vi "Communication Handler.vi"(8 "error in":errorcluster, 11 "Message Queues in":T1) -> (0 "error out":errorcluster)   [LabVIEW 2018]
uses:
  support/Message Queue/All Message Queues.ctl
  support/Message Queue/Message Cluster.ctl
  Real-Time/controls/Controller Data.ctl
  support/Message Queue/Enqueue Message (Single).vi
  support/Message Queue/Message Queue.lvlib
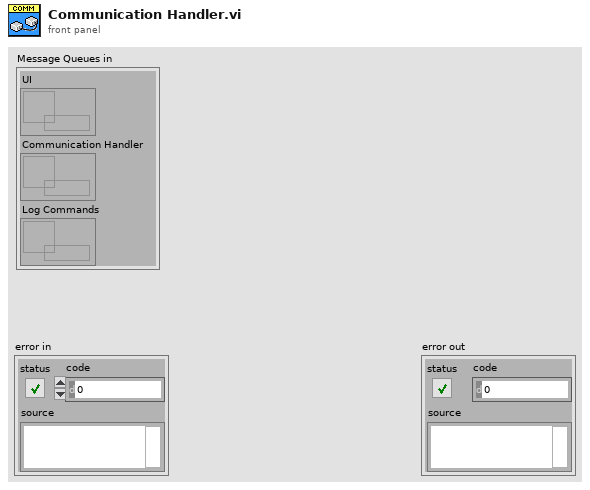
[diagram p1: front panel]
types:
  T1 = typedef "Message Queue.lvlib/All Message Queues.ctl" = cluster{"UI":refnum<queue>, "Communication Handler":refnum<queue>, "Log Commands":refnum<queue>}
  T2 = typedef "Controller Data.ctl" = cluster{"Closed Loop Enabled":bool, "Proportional valve 1":dbl, "Proportional valve 2":dbl, "Plant Control Variables":cluster{"Tank 1 Level":dbl, "Tank 2 Level":dbl, "Tank 3 Level":dbl, "Tank 4 Level":dbl, "Pump 1":dbl, "Pump 2":dbl}, "Setpoints":cluster{"Setpoint tank 1":dbl, "Setpoint tank 2":dbl}, "Controller":cluster{"A":dbl[][], "B":dbl[][], "C":dbl[][], "D":dbl[][]}}
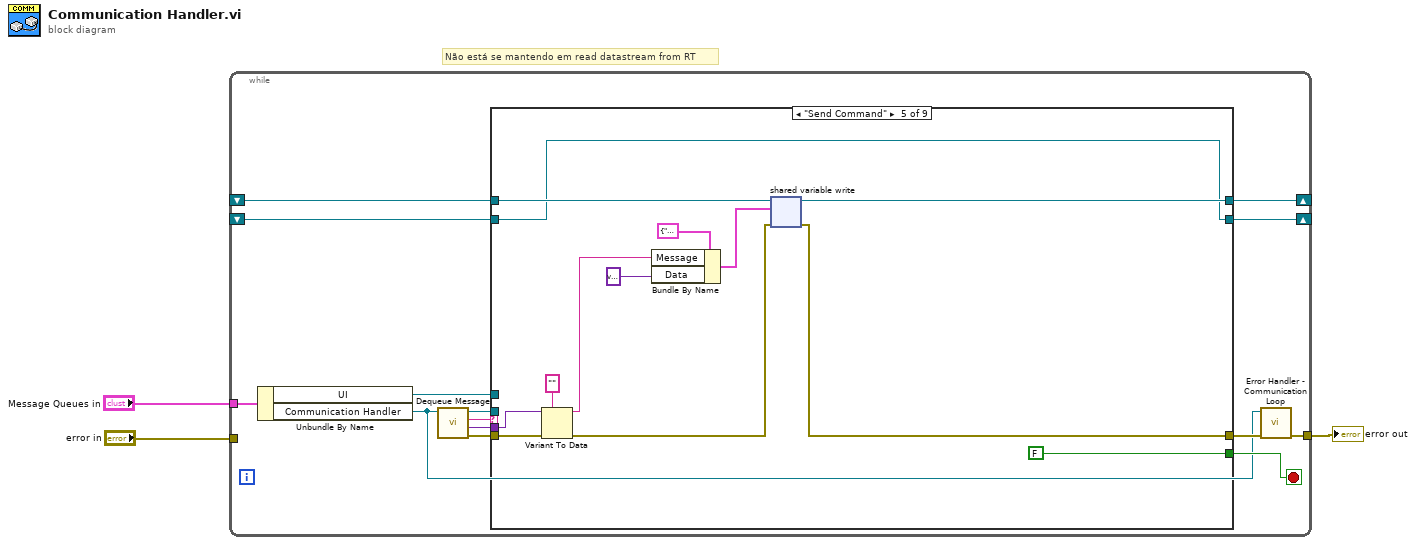
[diagram p0: block diagram]
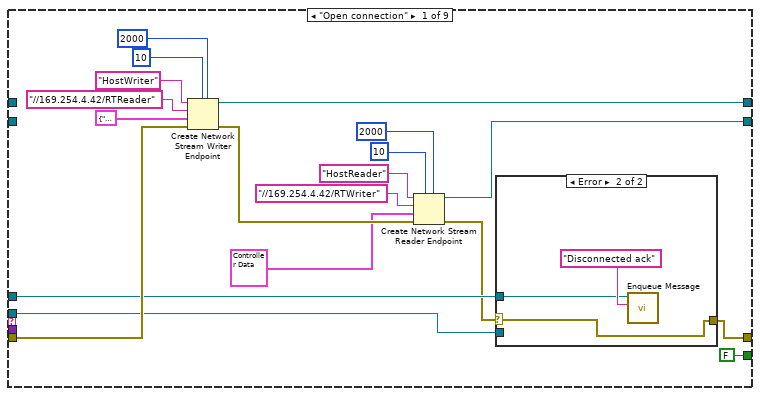
[diagram p2: hidden frame]
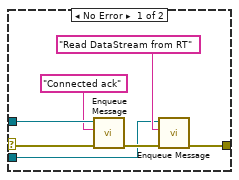
[diagram p3: hidden frame]
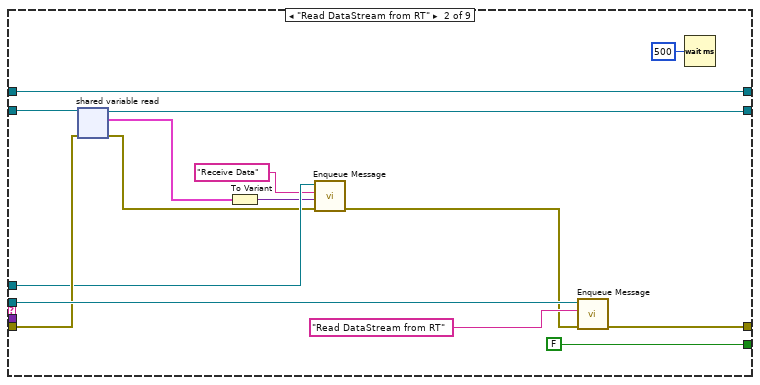
[diagram p4: hidden frame]
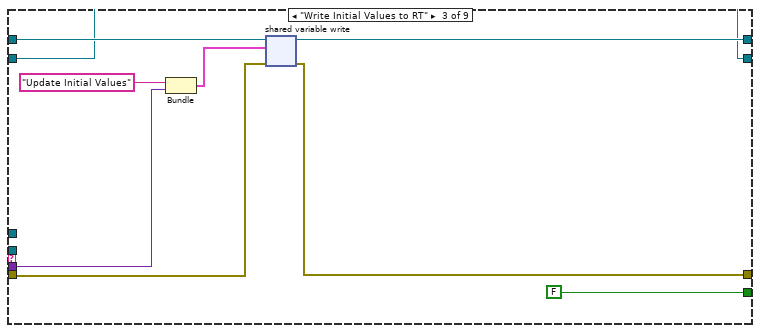
[diagram p5: hidden frame]
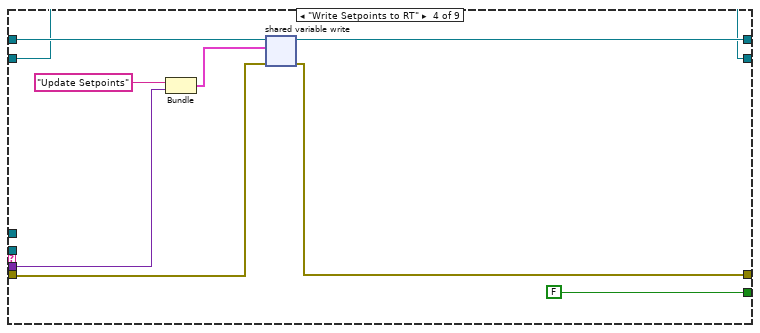
[diagram p6: hidden frame]
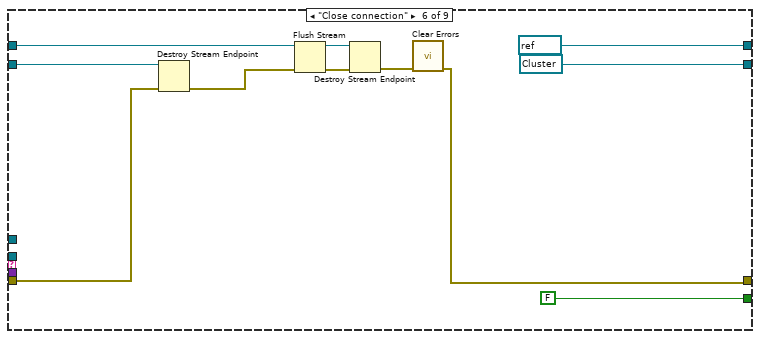
[diagram p7: hidden frame]
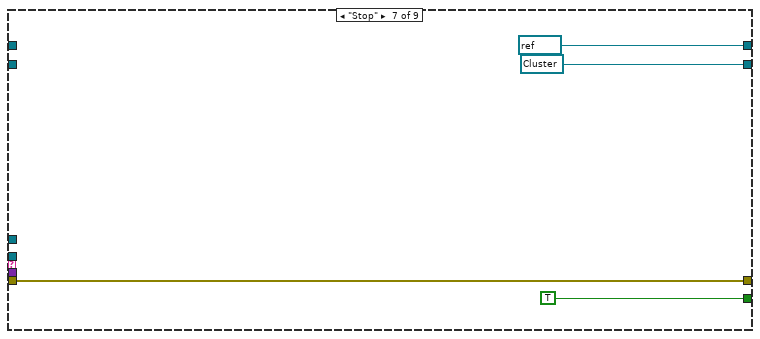
[diagram p8: hidden frame]
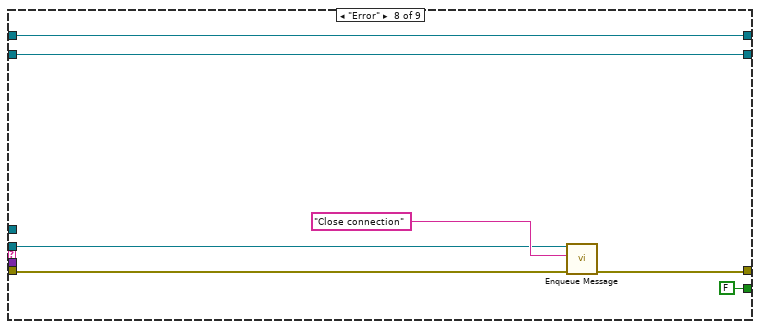
[diagram p9: hidden frame]
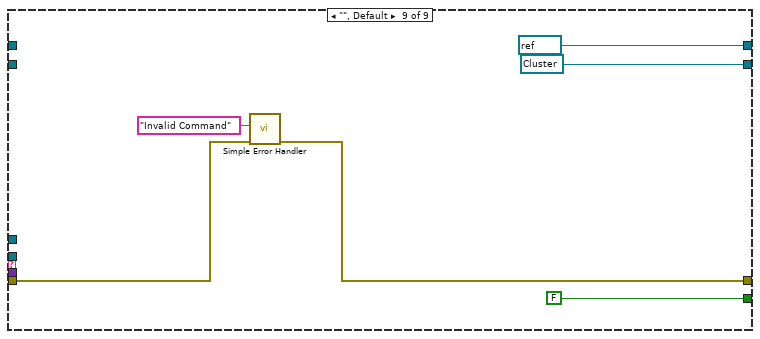
[diagram p10: hidden frame]
diagram:
  # "Não está se mantendo em read datastream from RT"
  n1 = while {
    tunnel: "Message Queues in" -> [w16]
    tunnel: [w6] -> w3
    tunnel: "error in" -> [_]
    shift-right: [w11] -> _
    shift-left: _ -> [w10]
    shift-right: [w4] -> _
    shift-left: _ -> [w9]
    stop <- w12 stop-if-true
    n2 = Unbundle By Name(w16) -> ("UI"=w15:refnum<queue>, "Communication Handler"=w5:refnum<queue>)
    n3 = call "Dequeue Message.vi"("Message Queue"=w5) -> ("error out"=w13:errorcluster, "Message Data"=w8:variant, "Message"=w17:string, "dup Message Queue"=w14:refnum<queue>)  [unwired: 7 in]
    n4 = case shown="\"Send Command\"" w17 {
      tunnel: w15 -> [w29 w56 _ _ _ _ _ _ _]
      tunnel: w14 -> [w20 w58 _ _ _ _ _ w112 _]
      tunnel: w13 -> [w30 w57 w66 w75 w86 w98 w105 w113 w120]
      tunnel: [w22 w60 w63 w72 w89 w94 w105 w109 w118] -> w7
      tunnel: [FALSE FALSE FALSE FALSE FALSE FALSE TRUE FALSE FALSE] -> w12
      tunnel: [w27 w51 w68 w77 w90 refnum<k21> refnum ("writer name") refnum<k21> refnum ("writer name") w111 refnum<k21> refnum ("writer name")] -> w11
      tunnel: w10 -> [_ w51 w69 w78 w91 w102 _ w111 _]
      tunnel: w9 -> [_ w49 w62 w71 w80 w96 _ w108 _]
      tunnel: w8 -> [_ _ w65 w74 w87 _ _ _ _]
      tunnel: [w18 w47 w62 w71 w80 refnum<k21> refnum ("writer name") refnum<k21> refnum ("writer name") w108 refnum<k21> refnum ("writer name")] -> w4
      frame "Open connection" {
        n5 = Create Network Stream Writer Endpoint(5:2000 ("timeout in ms (-1)"), 7:10 ("writer buffer size"), 8:w30, 9:cluster{string, variant} {"", variant}, 10:"//169.254.4.42/RTReader" ("writer url"), 11:"HostWriter" ("writer name")) -> (0:w31:errorcluster, 3:w27:refnum<k21>)  [unwired: 1 in]
        n6 = Create Network Stream Reader Endpoint(5:2000 ("timeout in ms (-1)"), 7:10 ("writer buffer size"), 8:w31, 9:T2 {"Closed Loop Enabled"=FALSE, "Proportional valve 1"=0.0, "Proportional valve 2"=0.0, "Plant Control Variables"={"Tank 1 Level"=0.0, "Tank 2 Level"=0.0, "Tank 3 Level"=0.0, "Tank 4 Level"=0.0, "Pump 1"=0.0, "Pump 2"=0.0}, "Setpoints"={"Setpoint tank 1"=0.0, "Setpoint tank 2"=0.0}, "Controller"={"A"=[[-4.94989, 0.0218181, -352.966, 23.8192, -3.10685, -0.000952287], [-0.0218181, -4.904857, 23.4819, -343.472, 0.000977323, -3.58066], [0.0389045, 0.0, -31.6573, 0.0287797, 0.0245405, 0.0], [0.0, 0.0381972, 0.0287797, -31.6573, 0.0, 0.0280468], [0.0, 0.0325383, 0.0240248, -0.0293675, -0.0245405, 0.0], [0.031831, 0.0, -0.0282058, 0.0, 0.0, 0.0]], "B"=[[28.0692, -23.9099], [-23.3912, 28.5852], [31.6468, -0.0287797], [-0.0287797, 31.6468], [-0.0282058, -0.0293675], [0.0282058, -0.0240214]], "C"=[[4.94989, 0.0218181, 314.896, 0.0907351, 3.10685, 0.000952287], [10.0218181, 4.90457, -0.0906726, 314.884, -0.000977323, 3.58066]], "D"=[[0.0, 0.0], [0.0, 0.0]]}} ("Cluster"), 10:"//169.254.4.42/RTWriter" ("writer url"), 11:"HostReader" ("writer name")) -> (0:w21:errorcluster, 3:w18:refnum<k21>)  [unwired: 1 in]
        n7 = case shown="Error" w21 {
          selector: w21 -> [w38 w44]
          tunnel: w29 -> [w43 w45]
          tunnel: [w41 w44] -> w22
          tunnel: w20 -> [w37 _]
          frame No Error {
            n8 = call-poly "Enqueue Message.vi"("error in (no error)"=w38, "Message"="Connected ack", "Message Queue"=w43) -> ("error out"=w42:errorcluster)  [unwired: 7 in, 1 out]
            n9 = call-poly "Enqueue Message.vi"("error in (no error)"=w42, "Message"="Read DataStream from RT", "Message Queue"=w37) -> ("error out"=w41:errorcluster)  [unwired: 7 in, 1 out]
          }
          frame Error {
            n10 = call-poly "Enqueue Message.vi"("Message"="Disconnected ack", "Message Queue"=w45) -> ()  [unwired: 8 in, 2 out]
          }
        }
      }
      frame "Read DataStream from RT" {
        n11 = shared-variable-read(w49, w57) -> (w47:refnum<k21>, w55:errorcluster, w48:T2)  [unwired: 1 in, 1 out]
        n12 = To Variant(anything=w48) -> (Variant=w53:variant)
        n13 = call-poly "Enqueue Message.vi"("error in (no error)"=w55, "Message Data"=w53, "Message"="Receive Data", "Message Queue"=w56) -> ("error out"=w52:errorcluster)  [unwired: 6 in, 1 out]
        n14 = call-poly "Enqueue Message.vi"("error in (no error)"=w52, "Message"="Read DataStream from RT", "Message Queue"=w58) -> ("error out"=w60:errorcluster)  [unwired: 7 in, 1 out]
        n15 = Wait (ms)(milliseconds to wait=u32 500) -> ()  [unwired: 1 out]
      }
      frame "Write Initial Values to RT" {
        n16 = Bundle("Update Initial Values", "Message Data"=w65) -> (w64:cluster{string, "Message Data":variant})  [unwired: 1 in]
        n17 = shared-variable-write(w69, w66, w64) -> (w68:refnum<k21>, w63:errorcluster)  [unwired: 1 in, 1 out]
      }
      frame "Write Setpoints to RT" {
        n18 = Bundle("Update Setpoints", "Message Data"=w74) -> (w73:cluster{string, "Message Data":variant})  [unwired: 1 in]
        n19 = shared-variable-write(w78, w75, w73) -> (w77:refnum<k21>, w72:errorcluster)  [unwired: 1 in, 1 out]
      }
      frame "Send Command" {
        n20 = Variant To Data(error in=w86, type="", Variant=w87) -> (data=w83:string, error out=w85:errorcluster)
        n21 = Bundle By Name(cluster=cluster{"Message":string, "Data":variant} {"Message"="", "Data"=variant}, "Message"=w83, "Data"=variant) -> (w92:cluster{"Message":string, "Data":variant})
        n22 = shared-variable-write(w91, w85, w92) -> (w90:refnum<k21>, w89:errorcluster)  [unwired: 1 in, 1 out]
      }
      frame "Close connection" {
        n23 = Destroy Stream Endpoint(8:w98, 11:w96) -> (0:w99:errorcluster)
        n24 = Flush Stream(8:w99, 11:w102) -> (0:w100:errorcluster, 3:w101:refnum<k21>)  [unwired: 2 in, 1 out]
        n25 = Destroy Stream Endpoint(8:w100, 11:w101) -> (0:w95:errorcluster)
        n26 = call <vilib>:"Clear Errors.vi"("error in (no error)"=w95) -> ("error out"=w94:errorcluster)  [unwired: 5 in, 1 out]
      }
      frame "Stop" {
      }
      frame "Error" {
        n27 = call-poly "Enqueue Message.vi"("error in (no error)"=w113, "Message"="Close connection", "Message Queue"=w112) -> ("error out"=w109:errorcluster)  [unwired: 7 in, 1 out]
      }
      frame "", Default {
        n28 = call <vilib>:"Simple Error Handler.vi"("error source (\" \")"="Invalid Command" ("error source (\" \")"), "error in (no error)"=w120) -> ("error out"=w118:errorcluster)  [unwired: 3 in, 4 out]
      }
    }
    n29 = call "Error Handler - Communication Loop.vi"("error in (no error)"=w7, "Message Queue"=w5) -> ("dup error in"=w6:errorcluster)  [unwired: 8 in, 1 out]
  }
  "error out" <- w3
